vi "MDF4 Add Channel Group.vi"(6 "Record ID":u64, 8 "Error In":errorcluster, 10 "Data Group Reference in":i64, 11 "MDF4 File Reference in":i64) -> (0 "Error Out":errorcluster, 1 "Channel Group Reference out":i64, 2 "Data Group Reference out":i64, 3 "MDF4 File Reference out":i64)   [LabVIEW 2019, in "MD4Logger Engine.lvlib"]
uses:
  MD4Logger Engine.lvlib
  <vilib>/Utility/error.llb/Error Cluster From Error Code.vi
  <vilib>/ErrorRing/Error Ring.xnode
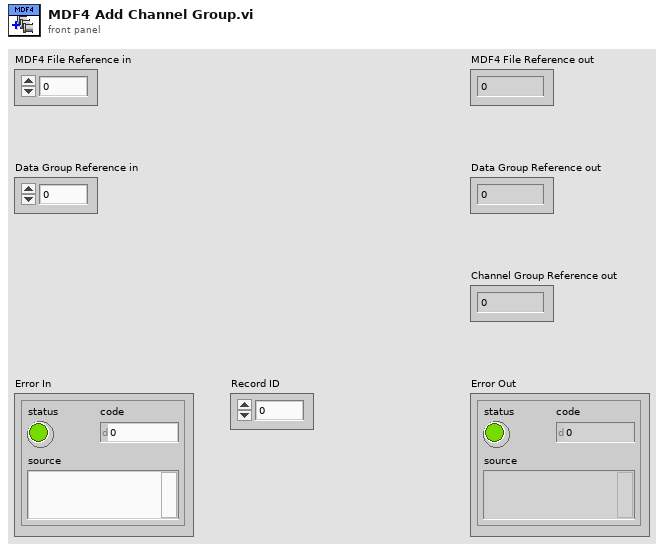
[diagram p1: front panel]
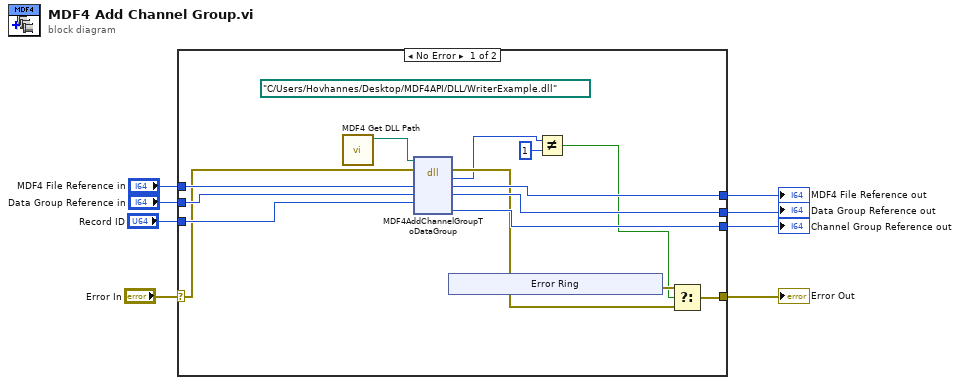
[diagram p0: block diagram]
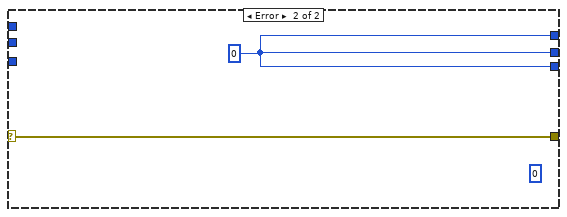
[diagram p2: hidden frame]
diagram:
  n1 = case shown="No Error" "Error In" {
    selector: "Error In" -> [w13 w29]
    tunnel: "MDF4 File Reference in" -> [w22 _]
    tunnel: [w14 w29] -> w6
    tunnel: [w21 w28] -> w5
    tunnel: [w20 w28] -> w4
    tunnel: "Data Group Reference in" -> [w19 _]
    tunnel: [w18 w28] -> w2
    tunnel: "Record ID" -> [w15 _]
    frame No Error {
      (unwired) path "C:/Users/Hovhannes/Desktop/MDF4API/DLL/WriterExample.dll" ("path in")
      n2 = call "MDF4 Get DLL Path.vi"() -> ("DLL Path Out"=w9:path)  [unwired: 11 in]
      n3 = dll-call lib="C:/Users/Hovhannes/Desktop/MDF4API/DLL/WriterExample.dll" fn="MDF4AddChannelGroupToDataGroup"(path in=w9, error in=w13, "m4"=w22, "dg"=w19, "rec_id"=w15) -> (error out=w16:errorcluster, "return type"=w11:i32, "m4"=w20:i64, "dg"=w21:i64, "cg"=w18:i64)  [unwired: 3 in, 1 out]
      n4 = xnode "Error Ring"() -> ("error out"=w17:errorcluster)
      n5 = Not Equal?(x=w11, y=1) -> (x != y?=w10:bool)
      n6 = Select(t=w17, s=w10, f=w16) -> (s? t:f=w14:errorcluster)
    }
    frame Error {
      (unwired) u32 0 ("byte_count")
      w28 = i64 0 ("m4")
    }
  }
  "Data Group Reference out" <- w5
  "Error Out" <- w6
  "MDF4 File Reference out" <- w4
  "Channel Group Reference out" <- w2
